vi "Name.vi"(8 "error in (no error)":errorcluster, 11 "Diagon Alley in":refnum<class "Diagon Alley.lvclass">) -> (0 "error out":errorcluster, 2 "Name":string, 3 "Diagon Alley out":refnum<class "Diagon Alley.lvclass">)   [LabVIEW 2020, in "Reversi.lvlib" / "Diagon Alley.lvclass"]
uses:
  Diagon Alley.lvclass
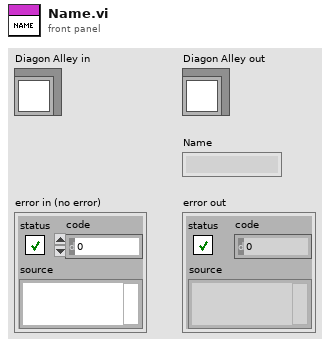
[diagram p1: front panel]
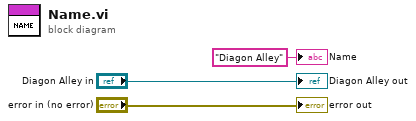
[diagram p0: block diagram]
diagram:
  "error out" <- "error in (no error)"
  "Diagon Alley out" <- "Diagon Alley in"
  "Name" <- "Diagon Alley" ("Name")
